vi "DMM FDVM Frequency_Period Individual.vi"() -> ()   [LabVIEW 2021]
uses:
  Signal Voltage Generation/Typedefs/Signal Generation Settings.ctl
  Signal Voltage Generation/Typedefs/Generation Types.ctl
  Signal Voltage Generation/Typedefs/Single Tone Settings.ctl
  Signal Voltage Generation/Typedefs/Waveform Type.ctl
  Signal Voltage Generation/Typedefs/Tone Settings.ctl
  DMM_Frequency Domain Measurement/Typedefs/Function Settings.ctl
  <instrlib>/niDMM/nidmm.llb/niDMM Resolution in Digits.ctl
  DMM_Frequency Domain Measurement/Typedefs/Timing & Trigger Settings.ctl
  <instrlib>/niDMM/nidmm.llb/niDMM Trigger.ctl
  <instrlib>/niDMM/nidmm.llb/niDMM Slope.ctl
  DMM_Frequency Domain Measurement/Typedefs/Measurement.ctl
  DMM_Frequency Domain Measurement/Typedefs/DMM Execution Settings.ctl
  Signal Voltage Generation/DAQ_Signal Voltage Generation.lvlib
  DMM_Frequency Domain Measurement/DMM_Frequency Domain Measurement.lvlib
panel:
  out "DMM Execution Settings":T1={"Absolute\nResolution"=7.5e-05, "Input Resistance\n(Ohm)"=1000000.0, "Digits\nResolution"=5.5, "Range"=15.0, "Minimum\nFrequency (Hz)"=20.0, "Aperture\nTime (s)"=0.14666666666666667, "Auto Range\nValue"=15.0, "Settle\nTime (s)"=0.5, "Function"=104} {"Function" items=["DC Volts"=1, "AC Volts"=2, "DC Current"=3, "AC Current"=4, "2-Wire Resistance"=5, "4-Wire Resistance"=101, "Frequency"=104, "Period"=105, "AC Volts DC Coupled"=1001, "Diode"=1002, "Waveform Voltage"=1003, "Waveform Current"=1004, "Capacitance"=1005, "Inductance"=1006, "Temperature"=108]; "Absolute\nResolution" format="%#_6p"; "Input Resistance\n(Ohm)" format="%#_6p"; "Range" format="%#_6p"; "Minimum\nFrequency (Hz)" format="%#_6p"; "Aperture\nTime (s)" format="%#_6p"; "Auto Range\nValue" format="%#_6p"; "Settle\nTime (s)" format="%#_6p"}
  out "Measurement":T2={"Measured Value"=99.99955026657287, "Out of Range"=FALSE, "Unit"="Hz", "Measurement"="99.9996Hz"} {"Measured Value" format="%^#_9e"}
  in  "Timing & Trigger Settings":T3={"Aperture Time (s)"=-1.0, "Settle Time (s)"=-1.0, "Trigger Settings"={"Trigger Delay (sec)"=-1.0, "Enable Trigger?"=FALSE, "Trigger Source"=enum."Immediate", "Slope"=enum."Rising Edge"}} caption="Timing and Trigger Settings" {"Trigger Settings"."Trigger Delay (sec)" format="%.4f"; "Aperture Time (s)" format="%#.6g"}
  in  "Function Settings":T6={"Resolution in Digits"=5.5, "Range and Function"=enum."Freq AC 5 V"} {"Resolution in Digits" items=["3 1/2"=3.5, "4 1/2"=4.5, "5 1/2"=5.5, "6 1/2"=6.5, "7 1/2"=7.5]}
  in  "Signal Generation Settings":T8={"Generation Type"=enum."Single Tone", "Generation Time (s)"=1.0, "Voltage Offset (v)"=1.0, "Single Tone Settings"={"Waveform Type"=enum."Square Wave", "Frequency (Hz)"=100.0, "Amplitude (V)"=1.0, "Duty Cycle (%)"=50.0}, "Multi Tone Settings"=[]} {"Voltage Offset (v)" format="%.2p"; "Generation Time (s)" format="%.2p"; "Multi Tone Settings"."Amplitude (V)" format="%.2p"; "Multi Tone Settings"."Frequency (Hz)" format="%.2p"; "Single Tone Settings"."Duty Cycle (%)" format="%.2p"; "Single Tone Settings"."Amplitude (V)" format="%.2p"; "Single Tone Settings"."Frequency (Hz)" format="%.2p"}
  in  "DMM Resource Name":refnum<k15>="DMM_4080"
  out "error out":errorcluster
  # "Frequency (Hz)"
  # "Amplitude (V)"
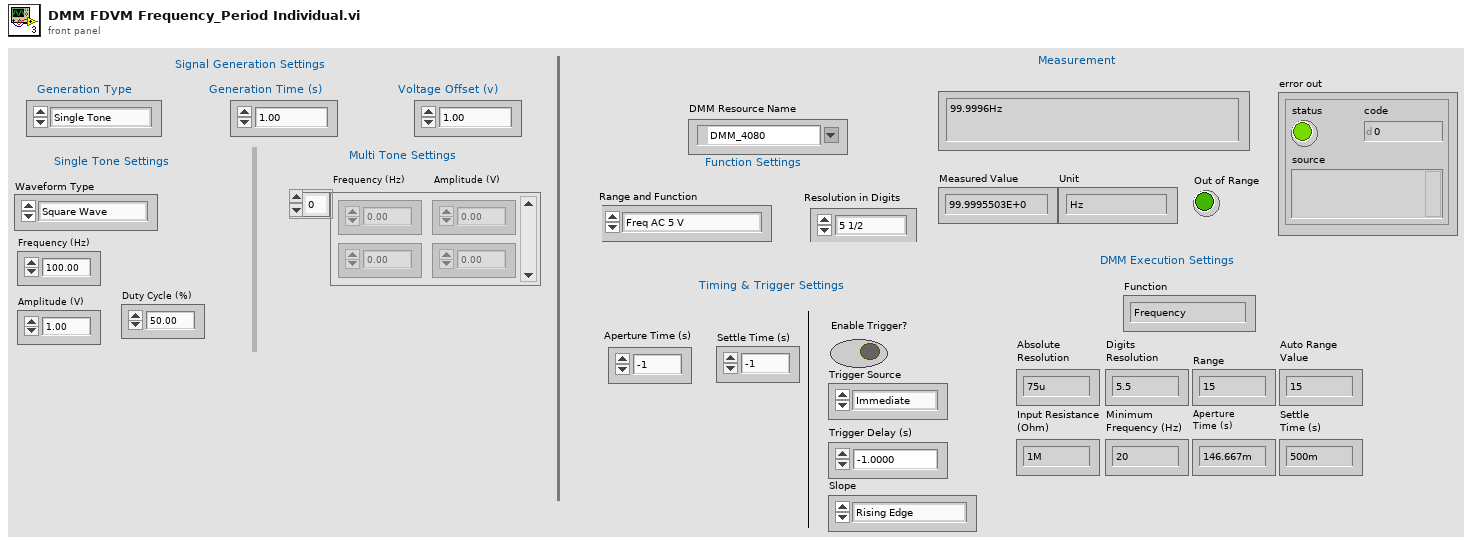
[diagram p1: front panel]
types:
  T1 = typedef "DMM_Frequency Domain Measurement.lvlib/DMM Execution Settings.ctl" = cluster{"Absolute\nResolution":dbl, "Input Resistance\n(Ohm)":dbl, "Digits\nResolution":dbl, "Range":dbl, "Minimum\nFrequency (Hz)":dbl, "Aperture\nTime (s)":dbl, "Auto Range\nValue":dbl, "Settle\nTime (s)":dbl, "Function":i32}
  T2 = typedef "DMM_Frequency Domain Measurement.lvlib/Measurement.ctl" = cluster{"Measured Value":dbl, "Out of Range":bool, "Unit":string, "Measurement":string}
  T3 = typedef "DMM_Frequency Domain Measurement.lvlib/Timing & Trigger Settings.ctl" = cluster{"Aperture Time (s)":dbl, "Settle Time (s)":dbl, "Trigger Settings":cluster{"Trigger Delay (sec)":dbl, "Enable Trigger?":bool, "Trigger Source":T4, "Slope":T5}}
  T4 = typedef "niDMM Trigger.ctl" = enum16{"Immediate", "External", "TTL 0", "TTL 1", "TTL 2", "TTL 3", "TTL 4", "TTL 5", "TTL 6", "Software", "TTL 7", "PXI Star", "LBR Trig 1", "Aux Trig 1"}
  T5 = typedef "niDMM Slope.ctl" = enum16{"Rising Edge", "Falling Edge"}
  T6 = typedef "DMM_Frequency Domain Measurement.lvlib/Function Settings.ctl" = cluster{"Resolution in Digits":T7, "Range and Function":enum16{"Frequency AC Auto Range", "Freq AC 50 mV", "Freq AC 500 mV", "Freq AC 5 V", "Freq AC 50 V", "Freq AC 300 V", "      ", "Period AC Auto Range", "Period AC 50 mV", "Period AC 500 mV", "Period AC 5 V", "Period AC 50 V", "Period AC 300 V"}}
  T7 = typedef "niDMM Resolution in Digits.ctl" = dbl
  T8 = typedef "DAQ_Signal Voltage Generation.lvlib/Signal Generation Settings.ctl" = cluster{"Generation Type":T9, "Generation Time (s)":dbl, "Voltage Offset (v)":dbl, "Single Tone Settings":T10, "Multi Tone Settings":T12[]}
  T9 = typedef "DAQ_Signal Voltage Generation.lvlib/Generation Types.ctl" = enum16{"Single Tone", "Multi Tone"}
  T10 = typedef "DAQ_Signal Voltage Generation.lvlib/Single Tone Settings.ctl" = cluster{"Waveform Type":T11, "Frequency (Hz)":dbl, "Amplitude (V)":dbl, "Duty Cycle (%)":dbl}
  T11 = typedef "DAQ_Signal Voltage Generation.lvlib/Waveform Type.ctl" = enum16{"Sine Wave", "Square Wave"}
  T12 = typedef "DAQ_Signal Voltage Generation.lvlib/Tone Settings.ctl" = cluster{"Frequency (Hz)":dbl, "Amplitude (V)":dbl}
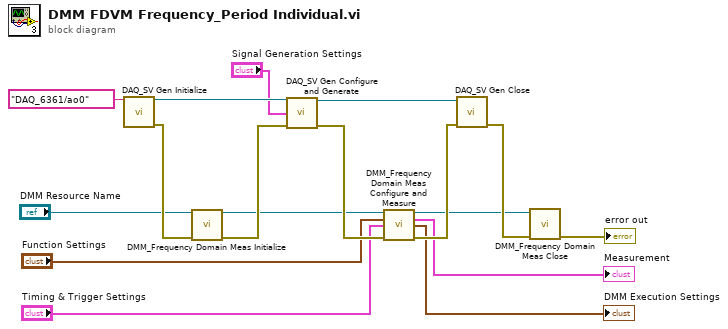
[diagram p0: block diagram]
diagram:
  n1 = call "DAQ_SV Gen Initialize.vi"("Physical Channels"=tag "DAQ_6361/ao0") -> ("DAQmx Task Out"=w11:refnum<k21>, "error out"=w17:errorcluster)  [unwired: 13 in]
  n2 = call "DMM_Frequency Domain Meas Initialize.vi"("DMM Resource Name"="DMM Resource Name", "error in"=w17) -> ("DMM Handle Out"=w9:refnum<k15>, "error out"=w16:errorcluster)  [unwired: 12 in]
  n3 = call "DAQ_SV Gen Configure and Generate.vi"("DAQmx Task In"=w11, "Signal Generation Settings"="Signal Generation Settings", "error in"=w16) -> ("DAQmx Task Out"=w10:refnum<k21>, "error out"=w15:errorcluster)  [unwired: 10 in, 1 out]
  n4 = call "DMM_Frequency Domain Meas Configure and Measure.vi"("DMM Handle In"=w9, "Function Settings"="Function Settings", "Timing & Trigger Settings"="Timing & Trigger Settings", "error in"=w15) -> ("DMM Handle Out"=w8:refnum<k15>, "Measurement"=→"Measurement":T2, "DMM Execution Settings"=→"DMM Execution Settings":T1, "error out"=w14:errorcluster)  [unwired: 8 in]
  n5 = call "DAQ_SV Gen Close.vi"("DAQmx Task In"=w10, "error in"=w14) -> ("error out"=w13:errorcluster)  [unwired: 13 in]
  n6 = call "DMM_Frequency Domain Meas Close.vi"("DMM Handle In"=w8, "error in"=w13) -> ("error out"=→"error out":errorcluster)  [unwired: 13 in]
